vi "HFRR ADV v04 new software.vi"() -> ()   [LabVIEW 2025] (continued)
              n1808 = String Subset(string=w2052, offset (0)=25, length (rest)=9 ("length (rest)")) -> (substring=w2057:string)
              n1809 = String Subset(string=w2052, offset (0)=45, length (rest)=9 ("length (rest)")) -> (substring=w2065:string)
              n1810 = String Subset(string=w2052, offset (0)=0, length (rest)=14 ("length (rest)")) -> (substring=w2080:string)
              n1811 = String Subset(string=w2052, offset (0)=15, length (rest)=9 ("length (rest)")) -> (substring=w2083:string)
              n1812 = String Subset(string=w2052, offset (0)=65, length (rest)=9 ("length (rest)")) -> (substring=w2069:string)
              n1813 = Fract/Exp String To Number(string=w2055) -> (number=w2051:dbl)  [unwired: 3 in, 1 out]
              n1814 = Fract/Exp String To Number(string=w2077) -> (number=w2075:dbl)  [unwired: 3 in, 1 out]
              n1815 = Fract/Exp String To Number(string=w2063) -> (number=w2060:dbl)  [unwired: 3 in, 1 out]
              n1816 = Fract/Exp String To Number(string=w2057) -> (number=w2056:dbl)  [unwired: 3 in, 1 out]
              n1817 = Fract/Exp String To Number(string=w2065) -> (number=w2064:dbl)  [unwired: 3 in, 1 out]
              n1818 = Fract/Exp String To Number(string=w2080) -> (number=w2076:dbl)  [unwired: 3 in, 1 out]
              n1819 = Fract/Exp String To Number(string=w2083) -> (number=w2074:dbl)  [unwired: 3 in, 1 out]
              n1820 = Fract/Exp String To Number(string=w2069) -> (number=w2072:dbl)  [unwired: 3 in, 1 out]
              n1821 = Add(x=w2072, y=0.0) -> (x+y=w2068:dbl)
            }
            n1822 = for {
              N: w1960 -> [_]
              tunnel: w1967 -> [w2015]
              tunnel: w1966 -> [w2014]
              tunnel: [w2004] -> w1920 mode=indexing
              tunnel: [w2003] -> w1913 mode=indexing
              tunnel: w1957 -> [_]
              tunnel: [w1992] -> w1918 mode=indexing
              tunnel: [w1997] -> w1915 mode=indexing
              tunnel: [w1993] -> w1905 mode=indexing
              tunnel: [w1988] -> w1880 mode=indexing
              tunnel: [w1984] -> w1861 mode=indexing
              tunnel: [w1979] -> w1821 mode=indexing
              (unwired) 1.0 ("x")
              (unwired) TRUE ("line mode (F)")
              n1823 = Read from Text File "Read File"(file (use dialog)=w2015, error in=w2014) -> (text=w1980:string)  [unwired: 2 in, 3 out]
              n1824 = local write "String 12"(w1980) -> ()
              n1825 = String Subset(string=w1980, offset (0)=85, length (rest)=9 ("length (rest)")) -> (substring=w1982:string)
              n1826 = String Subset(string=w1980, offset (0)=35, length (rest)=9 ("length (rest)")) -> (substring=w2005:string)
              n1827 = String Subset(string=w1980, offset (0)=55, length (rest)=9 ("length (rest)")) -> (substring=w1990:string)
              n1828 = String Subset(string=w1980, offset (0)=25, length (rest)=9 ("length (rest)")) -> (substring=w1986:string)
              n1829 = String Subset(string=w1980, offset (0)=45, length (rest)=9 ("length (rest)")) -> (substring=w1995:string)
              n1830 = String Subset(string=w1980, offset (0)=15, length (rest)=9 ("length (rest)")) -> (substring=w2011:string)
              n1831 = String Subset(string=w1980, offset (0)=0, length (rest)=14 ("length (rest)")) -> (substring=w2008:string)
              n1832 = String Subset(string=w1980, offset (0)=65, length (rest)=9 ("length (rest)")) -> (substring=w1998:string)
              n1833 = Fract/Exp String To Number(string=w1982) -> (number=w1979:dbl)  [unwired: 3 in, 1 out]
              n1834 = Fract/Exp String To Number(string=w2005) -> (number=w2003:dbl)  [unwired: 3 in, 1 out]
              n1835 = Fract/Exp String To Number(string=w1990) -> (number=w1988:dbl)  [unwired: 3 in, 1 out]
              n1836 = Fract/Exp String To Number(string=w1986) -> (number=w1984:dbl)  [unwired: 3 in, 1 out]
              n1837 = Fract/Exp String To Number(string=w1995) -> (number=w1993:dbl)  [unwired: 3 in, 1 out]
              n1838 = Fract/Exp String To Number(string=w2011) -> (number=w1992:dbl)  [unwired: 3 in, 1 out]
              n1839 = Fract/Exp String To Number(string=w2008) -> (number=w2004:dbl)  [unwired: 3 in, 1 out]
              n1840 = Fract/Exp String To Number(string=w1998) -> (number=w2001:dbl)  [unwired: 3 in, 1 out]
              n1841 = Add(x=w2001, y=0.0) -> (x+y=w1997:dbl)
            }
            n1842 = Delete From Array(array=w1863, index=0) -> (array with subset deleted=w1836:dbl[])  [unwired: 1 in, 1 out]
            n1843 = Delete From Array(array=w1926, index=0) -> (array with subset deleted=w1899:dbl[])  [unwired: 1 in, 1 out]
            n1844 = Delete From Array(array=w1906, index=0) -> (array with subset deleted=w1894:dbl[])  [unwired: 1 in, 1 out]
            n1845 = Delete From Array(array=w1924, index=0) -> (array with subset deleted=w1925:dbl[])  [unwired: 1 in, 1 out]
            n1846 = call-poly <vilib>:"Mean.vi"("X"=w1836) -> ("mean"=→"КОФ2 4":dbl)  [unwired: 1 out]
            n1847 = call-poly <vilib>:"Mean.vi"("X"=w1899) -> ("mean"=→"КОФ3":dbl)  [unwired: 1 out]
            n1848 = call-poly <vilib>:"Mean.vi"("X"=w1894) -> ("mean"=→"CP3":dbl)  [unwired: 1 out]
            n1849 = Delete From Array(array=w1888, index=0) -> (array with subset deleted=w1815:dbl[])  [unwired: 1 in, 1 out]
            n1850 = Delete From Array(array=w1827, index=0) -> (array with subset deleted=w1814:dbl[])  [unwired: 1 in, 1 out]
            n1851 = Delete From Array(array=w1867, index=0) -> (array with subset deleted=w1838:dbl[])  [unwired: 1 in, 1 out]
            n1852 = Delete From Array(array=w1945, index=0) -> (array with subset deleted=w1900:dbl[])  [unwired: 1 in, 1 out]
            n1853 = Delete From Array(array=w1911, index=0) -> (array with subset deleted=w1896:dbl[])  [unwired: 1 in, 1 out]
            "array w/ subset deleted" <- w1896
            n1854 = Delete From Array(array=w1942, index=0) -> (array with subset deleted=w1943:dbl[])  [unwired: 1 in, 1 out]
            n1855 = call-poly <vilib>:"Mean.vi"("X"=w1838) -> ("mean"=→"КОФ2 2":dbl)  [unwired: 1 out]
            n1856 = call-poly <vilib>:"Mean.vi"("X"=w1900) -> ("mean"=→"КОФ1":dbl)  [unwired: 1 out]
            n1857 = Bundle "Bundle"(w1815, w1814) -> (w1820:cluster{dbl[], dbl[]})  [unwired: 1 in]
            n1858 = Bundle "Bundle"(w1815, w1943) -> (w1807:cluster{dbl[], dbl[]})  [unwired: 1 in]
            n1859 = Delete From Array(array=w1822, index=0) -> (array with subset deleted=w1810:dbl[])  [unwired: 1 in, 1 out]
            n1860 = Delete From Array(array=w1823, index=0) -> (array with subset deleted=w1812:dbl[])  [unwired: 1 in, 1 out]
            n1861 = Delete From Array(array=w1933, index=0) -> (array with subset deleted=w1934:dbl[])  [unwired: 1 in, 1 out]
            n1862 = Delete From Array(array=w1821, index=0) -> (array with subset deleted=w1808:dbl[])  [unwired: 1 in, 1 out]
            n1863 = Delete From Array(array=w1915, index=0) -> (array with subset deleted=w1916:dbl[])  [unwired: 1 in, 1 out]
            n1864 = Delete From Array(array=w1940, index=0) -> (array with subset deleted=w1846:dbl[])  [unwired: 1 in, 1 out]
            n1865 = Delete From Array(array=w1886, index=0) -> (array with subset deleted=w1842:dbl[])  [unwired: 1 in, 1 out]
            n1866 = Delete From Array(array=w1922, index=0) -> (array with subset deleted=w1844:dbl[])  [unwired: 1 in, 1 out]
            n1867 = Delete From Array(array=w1882, index=0) -> (array with subset deleted=w1840:dbl[])  [unwired: 1 in, 1 out]
            n1868 = Delete From Array(array=w1931, index=0) -> (array with subset deleted=w1845:dbl[])  [unwired: 1 in, 1 out]
            n1869 = Delete From Array(array=w1884, index=0) -> (array with subset deleted=w1841:dbl[])  [unwired: 1 in, 1 out]
            n1870 = Delete From Array(array=w1865, index=0) -> (array with subset deleted=w1837:dbl[])  [unwired: 1 in, 1 out]
            n1871 = Delete From Array(array=w1909, index=0) -> (array with subset deleted=w1895:dbl[])  [unwired: 1 in, 1 out]
            n1872 = Delete From Array(array=w1936, index=0) -> (array with subset deleted=w1897:dbl[])  [unwired: 1 in, 1 out]
            n1873 = Delete From Array(array=w1913, index=0) -> (array with subset deleted=w1843:dbl[])  [unwired: 1 in, 1 out]
            n1874 = Delete From Array(array=w1880, index=0) -> (array with subset deleted=w1839:dbl[])  [unwired: 1 in, 1 out]
            n1875 = Delete From Array(array=w1861, index=0) -> (array with subset deleted=w1835:dbl[])  [unwired: 1 in, 1 out]
            n1876 = Delete From Array(array=w1905, index=0) -> (array with subset deleted=w1893:dbl[])  [unwired: 1 in, 1 out]
            n1877 = Delete From Array(array=w1918, index=0) -> (array with subset deleted=w1898:dbl[])  [unwired: 1 in, 1 out]
            n1878 = Delete From Array(array=w1928, index=0) -> (array with subset deleted=w1811:dbl[])  [unwired: 1 in, 1 out]
            n1879 = Delete From Array(array=w1938, index=0) -> (array with subset deleted=w1813:dbl[])  [unwired: 1 in, 1 out]
            n1880 = Delete From Array(array=w1920, index=0) -> (array with subset deleted=w1809:dbl[])  [unwired: 1 in, 1 out]
            n1881 = Bundle "Bundle"(w1815, w1846) -> (w1833:cluster{dbl[], dbl[]})  [unwired: 1 in]
            n1882 = Bundle "Bundle"(w1815, w1900) -> (w1834:cluster{dbl[], dbl[]})  [unwired: 1 in]
            n1883 = Bundle "Bundle"(w1846, w1842) -> (w1848:cluster{dbl[], dbl[]})  [unwired: 1 in]
            n1884 = Bundle "Bundle"(w1811, w1810) -> (w1818:cluster{dbl[], dbl[]})  [unwired: 1 in]
            n1885 = Bundle "Bundle"(w1844, w1840) -> (w1850:cluster{dbl[], dbl[]})  [unwired: 1 in]
            n1886 = Bundle "Bundle"(w1811, w1844) -> (w1954:cluster{dbl[], dbl[]})  [unwired: 1 in]
            n1887 = Bundle "Bundle"(w1811, w1840) -> (w1878:cluster{dbl[], dbl[]})  [unwired: 1 in]
            n1888 = Bundle "Bundle"(w1811, w1899) -> (w1964:cluster{dbl[], dbl[]})  [unwired: 1 in]
            n1889 = Bundle "Bundle"(w1811, w1894) -> (w1902:cluster{dbl[], dbl[]})  [unwired: 1 in]
            n1890 = Bundle "Bundle"(w1811, w1925) -> (w1949:cluster{dbl[], dbl[]})  [unwired: 1 in]
            n1891 = Bundle "Bundle"(w1845, w1841) -> (w1849:cluster{dbl[], dbl[]})  [unwired: 1 in]
            n1892 = Bundle "Bundle"(w1813, w1812) -> (w1819:cluster{dbl[], dbl[]})  [unwired: 1 in]
            n1893 = Bundle "Bundle"(w1813, w1845) -> (w1956:cluster{dbl[], dbl[]})  [unwired: 1 in]
            n1894 = Bundle "Bundle"(w1813, w1841) -> (w1879:cluster{dbl[], dbl[]})  [unwired: 1 in]
            n1895 = Bundle "Bundle"(w1813, w1895) -> (w1903:cluster{dbl[], dbl[]})  [unwired: 1 in]
            n1896 = Bundle "Bundle"(w1813, w1897) -> (w1965:cluster{dbl[], dbl[]})  [unwired: 1 in]
            n1897 = Bundle "Bundle"(w1813, w1934) -> (w1947:cluster{dbl[], dbl[]})  [unwired: 1 in]
            n1898 = Bundle "Bundle"(w1843, w1839) -> (w1851:cluster{dbl[], dbl[]})  [unwired: 1 in]
            n1899 = Bundle "Bundle"(w1809, w1808) -> (w1817:cluster{dbl[], dbl[]})  [unwired: 1 in]
            n1900 = Bundle "Bundle"(w1809, w1843) -> (w1955:cluster{dbl[], dbl[]})  [unwired: 1 in]
            n1901 = Bundle "Bundle"(w1809, w1839) -> (w1877:cluster{dbl[], dbl[]})  [unwired: 1 in]
            n1902 = Bundle "Bundle"(w1809, w1893) -> (w1901:cluster{dbl[], dbl[]})  [unwired: 1 in]
            n1903 = Bundle "Bundle"(w1809, w1898) -> (w1963:cluster{dbl[], dbl[]})  [unwired: 1 in]
            n1904 = Bundle "Bundle"(w1809, w1916) -> (w1948:cluster{dbl[], dbl[]})  [unwired: 1 in]
            n1905 = call-poly <vilib>:"Mean.vi"("X"=w1896) -> ("mean"=→"CP1":dbl)  [unwired: 1 out]
            n1906 = call-poly <vilib>:"Mean.vi"("X"=w1837) -> ("mean"=→"КОФ2 3":dbl)  [unwired: 1 out]
            n1907 = call-poly <vilib>:"Mean.vi"("X"=w1895) -> ("mean"=→"CP2":dbl)  [unwired: 1 out]
            n1908 = call-poly <vilib>:"Mean.vi"("X"=w1897) -> ("mean"=→"КОФ2":dbl)  [unwired: 1 out]
            n1909 = call-poly <vilib>:"Mean.vi"("X"=w1835) -> ("mean"=→"КОФ2 5":dbl)  [unwired: 1 out]
            n1910 = call-poly <vilib>:"Mean.vi"("X"=w1893) -> ("mean"=→"CP4":dbl)  [unwired: 1 out]
            n1911 = call-poly <vilib>:"Mean.vi"("X"=w1898) -> ("mean"=→"КОФ4":dbl)  [unwired: 1 out]
            n1912 = Bundle "Bundle"(w1815, w1842) -> (w1806:cluster{dbl[], dbl[]})  [unwired: 1 in]
            n1913 = Bundle "Bundle"(w1815, w1896) -> (w1829:cluster{dbl[], dbl[]})  [unwired: 1 in]
            n1914 = Build Array "Build Array"(w1806, w1829) -> (w1832:cluster{dbl[], dbl[]}[])
            "XY Graph 17" <- w1832
            n1915 = Build Array "Build Array"(w1820, w1819, w1818, w1817) -> (→"Frequency ( Hz )":cluster{dbl[], dbl[]}[])
            n1916 = Build Array "Build Array"(w1848, w1849, w1850, w1851) -> (→"Air Temp ( °C ) vs Humidity ( % RH )":cluster{dbl[], dbl[]}[])
            n1917 = Build Array "Build Array"(w1833, w1956, w1954, w1955) -> (→"Air Temperature  ( °C )":cluster{dbl[], dbl[]}[])
            n1918 = Build Array "Build Array"(w1806, w1879, w1878, w1877) -> (→"Humidity ( %RH )":cluster{dbl[], dbl[]}[])
            n1919 = Build Array "Build Array"(w1834, w1965, w1964, w1963) -> (→"Coefficient Of Friction":cluster{dbl[], dbl[]}[])
            n1920 = Build Array "Build Array"(w1829, w1903, w1902, w1901) -> (→"Sample Temperature ( °C )":cluster{dbl[], dbl[]}[])
            n1921 = Build Array "Build Array"(w1807, w1947, w1949, w1948) -> (→"XY Graph 13":cluster{dbl[], dbl[]}[])
            n1922 = Bundle "Bundle"(w1815, w1838) -> (w1860:cluster{dbl[], dbl[]})  [unwired: 1 in]
            n1923 = Bundle "Bundle"(w1811, w1836) -> (w1858:cluster{dbl[], dbl[]})  [unwired: 1 in]
            n1924 = Bundle "Bundle"(w1813, w1837) -> (w1859:cluster{dbl[], dbl[]})  [unwired: 1 in]
            n1925 = Bundle "Bundle"(w1809, w1835) -> (w1857:cluster{dbl[], dbl[]})  [unwired: 1 in]
            n1926 = Build Array "Build Array"(w1860, w1859, w1858, w1857) -> (→"Stroke ( mm )":cluster{dbl[], dbl[]}[])
            n1927 = local write "XY Graph 16"(w1832) -> ()
          }
          frame #2 {
          }
          frame #3 {
            n1928 = local write "Numeric 8"(0 ("Numeric 8")) -> ()
            n1929 = local write "Numeric 11"(0 ("Numeric 11")) -> ()
            n1930 = local write "Numeric 12"(0 ("Numeric 12")) -> ()
            n1931 = local write "Numeric 13"(0 ("Numeric 13")) -> ()
            n1932 = property on="OPEN" class="Bool (strict)"("Visible"=TRUE) -> ()  [unwired: 2 in, 2 out]
            n1933 = local read "String Control 2"() -> (w2132:string)
            n1934 = local read "String Control 4"() -> (w2131:string)
            n1935 = local read "String Control 6"() -> (w2130:string)
            n1936 = local read "String Control 8"() -> (w2129:string)
            n1937 = Match Pattern(string=w2132, regular expression="Samples / cycle :- ") -> (after substring=w2146:string)  [unwired: 1 in, 3 out]
            n1938 = Match Pattern(string=w2132, regular expression="Frequency :- ") -> (after substring=w2165:string)  [unwired: 1 in, 3 out]
            n1939 = Match Pattern(string=w2131, regular expression="Samples / cycle :- ") -> (after substring=w2142:string)  [unwired: 1 in, 3 out]
            n1940 = Match Pattern(string=w2131, regular expression="Frequency :- ") -> (after substring=w2160:string)  [unwired: 1 in, 3 out]
            n1941 = Match Pattern(string=w2130, regular expression="Samples / cycle :- ") -> (after substring=w2138:string)  [unwired: 1 in, 3 out]
            n1942 = Match Pattern(string=w2130, regular expression="Frequency :- ") -> (after substring=w2155:string)  [unwired: 1 in, 3 out]
            n1943 = Match Pattern(string=w2129, regular expression="Samples / cycle :- ") -> (after substring=w2134:string)  [unwired: 1 in, 3 out]
            n1944 = Match Pattern(string=w2129, regular expression="Frequency :- ") -> (after substring=w2150:string)  [unwired: 1 in, 3 out]
            n1945 = String Subset(string=w2146, length (rest)=6 ("length (rest)")) -> (substring=w2148:string)  [unwired: 1 in]
            n1946 = String Subset(string=w2165, length (rest)=9 ("length (rest)")) -> (substring=w2167:string)  [unwired: 1 in]
            n1947 = String Subset(string=w2142, length (rest)=6 ("length (rest)")) -> (substring=w2144:string)  [unwired: 1 in]
            n1948 = String Subset(string=w2160, length (rest)=9 ("length (rest)")) -> (substring=w2162:string)  [unwired: 1 in]
            n1949 = String Subset(string=w2138, length (rest)=6 ("length (rest)")) -> (substring=w2140:string)  [unwired: 1 in]
            n1950 = String Subset(string=w2155, length (rest)=9 ("length (rest)")) -> (substring=w2157:string)  [unwired: 1 in]
            n1951 = String Subset(string=w2134, length (rest)=6 ("length (rest)")) -> (substring=w2136:string)  [unwired: 1 in]
            n1952 = String Subset(string=w2150, length (rest)=9 ("length (rest)")) -> (substring=w2152:string)  [unwired: 1 in]
            n1953 = Fract/Exp String To Number(string=w2148) -> (number=w2128:dbl)  [unwired: 3 in, 1 out]
            n1954 = Fract/Exp String To Number(string=w2167) -> (number=w2168:dbl)  [unwired: 3 in, 1 out]
            n1955 = Fract/Exp String To Number(string=w2144) -> (number=w2127:dbl)  [unwired: 3 in, 1 out]
            n1956 = Fract/Exp String To Number(string=w2162) -> (number=w2163:dbl)  [unwired: 3 in, 1 out]
            n1957 = Fract/Exp String To Number(string=w2140) -> (number=w2126:dbl)  [unwired: 3 in, 1 out]
            n1958 = Fract/Exp String To Number(string=w2157) -> (number=w2158:dbl)  [unwired: 3 in, 1 out]
            n1959 = Fract/Exp String To Number(string=w2136) -> (number=w2125:dbl)  [unwired: 3 in, 1 out]
            n1960 = Fract/Exp String To Number(string=w2152) -> (number=w2153:dbl)  [unwired: 3 in, 1 out]
            n1961 = local write "sample1"(w2128) -> ()
            n1962 = local write "freq1"(w2168) -> ()
            n1963 = local write "sample2"(w2127) -> ()
            n1964 = local write "freq2"(w2163) -> ()
            n1965 = local write "sample3"(w2126) -> ()
            n1966 = local write "freq3"(w2158) -> ()
            n1967 = local write "sample4"(w2125) -> ()
            n1968 = local write "freq 4"(w2153) -> ()
          }
        }
      }
    }
    n1969 = case shown="True" w1617 {
      selector: w1617 -> [_ w1745]
      frame False {
      }
      frame True {
        n1970 = Not(x=w1745) -> (.not. x?=w1741:bool)
        n1971 = local write "service 3"(w1741) -> ()
        n1972 = local write "OPEN 6"(w1741) -> ()
        n1973 = call <vilib>:"System Exec.vi"("wait until completion? (T)"=TRUE, "command line"="C:\\LAB-IQ\\Scar View.exe") -> ("error out"=→"error out 5":errorcluster)  [unwired: 6 in, 3 out]
      }
    }
    n1974 = case shown="\"Acquire\", Default" w1628 {
      frame "Acquire", Default {
        w2641 = 0.2 ("y")
        w2646 = 1.0 ("y")
        w2647 = 0.8 ("y")
        # "Elapsed time\ncof\nstroke\nAir temp\nTemp\nHumidity"
        n1975 = disable-structure shown="Disabled" {
          frame Disabled {
            n1976 = local read "Flag"() -> (w2664:dbl)
            n1977 = local read "RUN"() -> (w2661:bool)
            n1978 = Not(x=w2661) -> (.not. x?=w2660:bool)
            n1979 = Equal?(x=w2664, y=10.0) -> (x = y?=w2662:bool)
            n1980 = And(x=w2662, y=w2660) -> (x .and. y?=w2659:bool)
            n1981 = case shown="True" w2659 {
              frame False {
              }
              frame True {
                w2665 = FALSE ("Heater Button")
                n1982 = local write "Humidity"(w2665) -> ()
                n1983 = local write "Heater Button"(w2665) -> ()
              }
            }
          }
          frame Enabled {
          }
        }
        n1984 = disable-structure shown="Disabled" {
          frame Disabled {
            n1985 = case shown="True" {
              selector: _ -> [_ _]
              frame False {
              }
              frame True {
                w2756 = TRUE ("Heater")
                n1986 = local write "Humidity"(w2756) -> ()
                n1987 = local write "Heater Button"(w2756) -> ()
                n1988 = local read "TEST STANDARD"() -> (w2759:T3)
                n1989 = local read "TEST STANDARD"() -> (w2754:T3)
                n1990 = Equal?(x=w2759, y=enum16{"ASTM D6079", "ISO 12156", "Custom"}."ISO 12156" ("Test Standard")) -> (x = y?=w2757:bool)
                n1991 = Equal?(x=w2754, y=enum16{"ASTM D6079", "ISO 12156", "Custom"}."ASTM D6079" ("Test Standard")) -> (x = y?=w2753:bool)
                n1992 = case shown="True" w2757 {
                  frame False {
                  }
                  frame True {
                    n1993 = local write "Heater"(TRUE ("Heater")) -> ()
                    n1994 = local write "airtempflg"(FALSE ("airtempflg")) -> ()
                  }
                }
                n1995 = case shown="True" w2753 {
                  frame False {
                  }
                  frame True {
                    n1996 = local write "Heater"(FALSE ("Heater")) -> ()
                    n1997 = local write "airtempflg"(TRUE ("airtempflg")) -> ()
                  }
                }
              }
            }
          }
          frame Enabled {
          }
        }
        n1998 = stacked-sequence {
          frame #0 {
            n1999 = case shown="True" "RST FF" {
              frame False {
              }
              frame True {
                w2822 = 0.0 ("X Scale.Range:Maximum")
                n2000 = property on="Frictional Force ( N )" class="WFChart (strict)"("XScale.Maximum"=600.0 ("X Scale.Range:Maximum"), "XScale.Minimum"=w2822, "YScale.Maximum"=10.0 ("Y Scale.Range:Maximum"), "YScale.Minimum"=w2822) -> ()  [unwired: 2 in, 2 out]
              }
            }
          }
          frame #1 {
            n2001 = case shown="True" "RST TEMP" {
              frame False {
              }
              frame True {
                n2002 = property on="Temperature ( Deg C )" class="WFChart (strict)"("XScale.Minimum"=0.0 ("X Scale.Range:Minimum"), "XScale.Maximum"=600.0 ("X Scale.Range:Maximum"), "YScale.Minimum"=0.0 ("Y Scale.Range:Minimum"), "YScale.Maximum"=100.0 ("Y Scale.Range:Maximum")) -> ()  [unwired: 2 in, 2 out]
              }
            }
          }
          frame #2 {
            n2003 = case shown="True" "RSTCOF" {
              frame False {
              }
              frame True {
                n2004 = property on="Coefficient of Friction" class="WFChart (strict)"("XScale.Minimum"=0.0 ("X Scale.Range:Minimum"), "XScale.Maximum"=600.0 ("X Scale.Range:Maximum"), "YScale.Maximum"=1.0 ("X Scale.Range:Minimum"), "YScale.Minimum"=0.0 ("X Scale.Range:Minimum")) -> ()  [unwired: 2 in, 2 out]
              }
            }
          }
          frame #3 {
            n2005 = case shown="True" "RSTCOF 2" {
              frame False {
              }
              frame True {
                (unwired) 100.0 ("Y Scale.Range:Maximum")
                (unwired) 0.0 ("Y Scale.Range:Minimum")
                (unwired) 600.0 ("X Scale.Range:Maximum")
                (unwired) 0.0 ("X Scale.Range:Minimum")
              }
            }
          }
          frame #4 {
            n2006 = case shown="True" "RSTCOF 3" {
              frame False {
              }
              frame True {
                n2007 = property on="Electrical Contact Resistance ( % )" class="WFChart (strict)"("XScale.Minimum"=0.0 ("X Scale.Range:Minimum"), "XScale.Maximum"=600.0 ("X Scale.Range:Maximum"), "YScale.Minimum"=0.0 ("Y Scale.Range:Minimum"), "YScale.Maximum"=100.0 ("Y Scale.Range:Maximum")) -> ()  [unwired: 2 in, 2 out]
              }
            }
          }
        }
        n2008 = disable-structure shown="Disabled" {
          frame Disabled {
            n2009 = case shown="True" {
              selector: _ -> [_ _]
              frame False {
              }
              frame True {
                n2010 = local read "zflag 2"() -> (w2723:dbl)
                n2011 = local read "yflag"() -> (w2725:dbl)
                n2012 = Equal?(x=w2725, y=2.0 ("tflag")) -> (x = y?=w2727:bool)
                n2013 = Equal?(x=w2723, y=3.0 ("tflag")) -> (x = y?=w2726:bool)
                n2014 = And(x=w2727, y=w2726) -> (x .and. y?=w2721:bool)
                n2015 = case shown="True" w2721 {
                  frame False {
                  }
                  frame True {
                    w2752 = 0.0 ("zflag")
                    n2016 = local write "zflag"(w2752) -> ()
                    n2017 = local write "zflag 2"(w2752) -> ()
                    n2018 = Delete(path (use dialog)=path "C:/LAB-IQ-NXT/WO 2449 TT.sig" ("file path (dialog if empty)")) -> (deleted path=w2751:path)  [unwired: 4 in, 2 out]
                    n2019 = Delete(path (use dialog)=path "C:/LAB-IQ-NXT/WO 2449 TRH.sig" ("file path (dialog if empty)")) -> (deleted path=w2746:path)  [unwired: 4 in, 2 out]
                    n2020 = local read "SEN.RUN HRS"() -> (w2738:dbl)
                    n2021 = local read "SENSOR TIME"() -> (w2736:dbl)
                    n2022 = call <vilib>:"compatOverwrite.vi"("overwrite (F)"=TRUE) -> ("overwrite?"=w2728:T23)
                    n2023 = call <vilib>:"compatOverwrite.vi"("overwrite (F)"=TRUE) -> ("overwrite?"=w2732:T23)
                    n2024 = local read "Total No. of Tests"() -> (w2739:dbl)
                    n2025 = Add(x=w2736, y=w2738) -> (x+y=w2737:dbl)
                    "SEN.RUN HRS" <- w2737
                    n2026 = Open/Create/Replace File(file path (use dialog)=w2751, operation (0:open)=w2728) -> (refnum out=w2729:refnum<file>, error out=w2730:errorcluster)  [unwired: 4 in, 1 out]
                    n2027 = Open/Create/Replace File(file path (use dialog)=w2746, operation (0:open)=w2732) -> (refnum out=w2733:refnum<file>, error out=w2734:errorcluster)  [unwired: 4 in, 1 out]
                    n2028 = Deny Access(4:w2730, 6:T21."deny none" ("deny mode (2)"), 7:w2729) -> (3:w2750:refnum<file>)  [unwired: 1 out]
                    n2029 = Deny Access(4:w2734, 6:T21."deny none" ("deny mode (2)"), 7:w2733) -> (3:w2742:refnum<file>)  [unwired: 1 out]
                    n2030 = Number To Decimal String(number=w2739) -> (decimal integer string=w2747:string)  [unwired: 1 in]
                    n2031 = Number To Decimal String(number=w2737) -> (decimal integer string=w2743:string)  [unwired: 1 in]
                    n2032 = Write to Binary File(file (use dialog)=w2750, data=w2747, 5:FALSE ("prepend array or string size? (T)")) -> ()  [unwired: 3 in, 3 out]
                    n2033 = Write to Binary File(file (use dialog)=w2742, data=w2743, 5:FALSE ("prepend array or string size? (T)")) -> ()  [unwired: 3 in, 3 out]
                  }
                }
              }
            }
          }
          frame Enabled {
          }
        }
        n2034 = local read "RUN"() -> (w2650:bool)
        n2035 = local read "run replace"() -> (w2654:bool)
        n2036 = local read "run replace"() -> (w2653:bool)
        n2037 = case shown="True" w2650 {
          frame False {
            n2038 = local write "run replace"(FALSE ("run replace")) -> ()
          }
          frame True {
            "run replace" <- TRUE ("run replace")
          }
        }
        n2039 = local read "RUN"() -> (w2658:bool)
        n2040 = local read "Set Temp"() -> (w2620:dbl)
        n2041 = local read "SetTemp"() -> (w2622:dbl)
        n2042 = case shown="False" w2658 {
          tunnel: [FALSE ("TEST RUNNING") TRUE ("TEST RUNNING")] -> w2657
          frame False {
            w2841 = 0.0 ("Flag")
            n2043 = local write "Elapsed time"(0.0 ("elapsedtime")) -> ()
            n2044 = local write "Time Remaining"(w2841) -> ()
            n2045 = local write "Flag"(w2841) -> ()
            n2046 = local write "Remaining Time"(w2841) -> ()
          }
          frame True {
            n2047 = local write "Flag"(10.0 ("Flag")) -> ()
          }
        }
        n2048 = case shown="False" w2654 {
          frame False {
            n2049 = local read "zflag"() -> (→"zflag 2":dbl)
            n2050 = local write "yflag"(2.0 ("tflag")) -> ()
            n2051 = local write "FLAG 4"(0.0 ("FLAG")) -> ()
          }
          frame True {
            n2052 = local write "yflag"(1.0 ("tflag")) -> ()
            n2053 = local write "zflag"(3.0 ("zflag")) -> ()
          }
        }
        n2054 = local read "acq 2"() -> (w2652:bool)
        n2055 = local read "AIR TEMP"() -> (w2615:dbl)
        n2056 = local read "Amb temp"() -> (w2619:dbl)
        n2057 = case shown="True" "Save & Continue" {
          frame False {
          }
          frame True {
            "acq 2" <- TRUE ("acq 2")
          }
        }
        n2058 = local read "Set Rh"() -> (w2621:dbl)
        n2059 = Add(x=w2622, y=w2647) -> (x+y=w2648:dbl)
        n2060 = Subtract(x=w2622, y=w2647) -> (x-y=w2649:dbl)
        n2061 = Add(x=w2620, y=w2641) -> (x+y=w2642:dbl)
        n2062 = Subtract(x=w2620, y=w2641) -> (x-y=w2643:dbl)
        n2063 = And(x=w2652, y=w2653) -> (x .and. y?=w2651:bool)
        n2064 = Greater Or Equal?(x=w2615, y=15.0) -> (x >= y?=w2616:bool)
        "powstat" <- w2616
        n2065 = local read "Humidity ( %RH )"() -> (w2618:dbl)
        n2066 = case shown="True" "Save & Continue" {
          frame False {
          }
          frame True {
            n2067 = while {
              tunnel: "0123456789abcdefghijklmnopqrstuvwxyzABCDEFGHIJKLMNOPQRSTUVWXYZ" ("string 2") -> [w2812]
              shift-right: [w2810] -> w2805
              shift-left: "" -> [w2809]
              i -> [w2819]
              stop <- w2818 stop-if-true
              n2068 = Random Number (0-1)() -> (number: 0 to 1=w2813:dbl)
              n2069 = Multiply(x=w2813, y=62.0) -> (x*y=w2815:dbl)
              n2070 = Decrement(x="Length") -> (x-1=w2808:i16)
              n2071 = To Word Integer(number=w2815) -> (16bit integer=w2816:i16)
              n2072 = String Subset(string=w2812, offset (0)=w2816, length (rest)=1 ("length (rest)")) -> (substring=w2811:string)
              n2073 = Greater Or Equal?(x=w2819, y=w2808) -> (x >= y?=w2818:bool)
              n2074 = Concatenate Strings(w2811, w2809) -> (w2810:string)
            }
            n2075 = local write "UUID"(w2805) -> ()
          }
        }
        n2076 = In Range and Coerce(upper limit=w2648, x=w2619, lower limit=w2649) -> (In Range?=w2638:bool)  [unwired: 1 out]
        n2077 = Add(x=w2621, y=w2646) -> (x+y=w2645:dbl)
        n2078 = Subtract(x=w2621, y=w2646) -> (x-y=w2644:dbl)
        n2079 = local read "TEMP"() -> (w2617:dbl)
        n2080 = case shown="True" "Save & Continue" {
          frame False {
          }
          frame True {
            n2081 = local read "Operator ID"() -> (w3116:string)
            n2082 = local read "FILE"() -> (w3122:string)
            n2083 = String Length(string=w3122) -> (length=w3120:i32)
            n2084 = String Length(string=w3116) -> (length=w3117:i32)
            n2085 = Greater?(x=w3120, y=0) -> (0:w3119:bool)
            n2086 = Greater?(x=w3117, y=0) -> (0:w3115:bool)
            n2087 = And(x=w3119, y=w3115) -> (x .and. y?=w3114:bool)
            n2088 = case shown="True" w3114 {
              frame False {
                n2089 = stacked-sequence {
                  frame #0 {
                    n2090 = One Button Dialog(message="Please Enter a File Name and Operator ID to save data !", button name ("OK")="Ok") -> ()  [unwired: 1 out]
                  }
                  frame #1 {
                    n2091 = local write "Save & Continue"(FALSE ("OK Button")) -> ()
                  }
                }
                n2092 = local write "Save & Continue"(FALSE ("OK Button")) -> ()
              }
              frame True {
                n2093 = stacked-sequence {
                  frame #0 {
                    n2094 = local read "FILE"() -> (w3128:string)
                    n2095 = call "file check.vi"("file name in"=w3128) -> ("file name out"=w3127:string)  [unwired: 9 in, 1 out]
                    n2096 = call <vilib>:"Application Directory.vi"() -> ("Application Directory"=w3138:path)
                    n2097 = Build Path(base path=w3138, name or relative path="data") -> (appended path=w3137:path)
                    n2098 = call <vilib>:"Trim Whitespace.vi"("string"=w3127) -> ("trimmed string"=w3135:string)  [unwired: 1 in]
                    n2099 = call <vilib>:"Trim Whitespace.vi"("string"=w3127) -> ("trimmed string"=w3136:string)  [unwired: 1 in]
                    n2100 = List Folder(path=w3137) -> (folder names=w3133:string[])  [unwired: 3 in, 3 out]
                    n2101 = Match Pattern(string=w3135, regular expression="_(") -> (before substring=w3132:string)  [unwired: 1 in, 3 out]
                    n2102 = for {
                      tunnel: w3133 -> [w3147] mode=indexing
                      tunnel: w3132 -> [w3145]
                      shift-right: [w3143] -> w3130
                      shift-left: bool[] [] -> [w3144]
                      n2103 = Match Pattern(string=w3147, regular expression="_(") -> (before substring=w3146:string)  [unwired: 1 in, 3 out]
                      n2104 = Equal?(x=w3146, y=w3145) -> (x = y?=w3142:bool)
                      n2105 = case shown="True" w3142 {
                        tunnel: w3142 -> [_ w3150]
                        tunnel: w3144 -> [w3149 w3152]
                        tunnel: [w3149 w3151] -> w3143
                        frame False {
                        }
                        frame True {
                          n2106 = Insert Into Array(array=w3152, new element=w3150) -> (w3151:bool[])  [unwired: 1 in]
                        }
                      }
                    }
                    n2107 = Equal?(x=w3133, y=w3132) -> (x = y?=w3141:bool[])
                    n2108 = Or Array Elements(Boolean array=w3141) -> (logical OR=w3140:bool)
                    n2109 = Array Size(array=w3130) -> (size(s)=w3129:i32)
                    n2110 = case shown="True" w3140 {
                      tunnel: w3136 -> [_ w3160]
                      tunnel: w3129 -> [_ w3153]
                      frame False {
                      }
                      frame True {
                        n2111 = Number To Decimal String(number=w3153) -> (decimal integer string=w3156:string)  [unwired: 1 in]
                        n2112 = Search/Split String(string=w3160, search string/char (-)="_(" ("regular expression")) -> (substring before match=w3158:string)  [unwired: 1 in, 2 out]
                        n2113 = Concatenate Strings(w3158, "_(" ("regular expression"), w3156, ")" ("regular expression")) -> (w3154:string)
                        n2114 = local write "FILE"(w3154) -> ()
                      }
                    }
                  }
                  frame #1 {
                    w3162 = 0.0
                    w3175 = cluster{"y":dbl, dbl, "y":dbl}[] [] ("History Data")
                    w3176 = FALSE ("Heater Button")
                    (unwired) ")!" ("string")
                    (unwired) ")" ("string")
                    w3174 = dbl[] [] ("History Data")
                    w3180 = "\r"
                    # "C:\\WinDucom\\Data\\"
                    # "C:\\LAB-IQ-NXT\\data"
                    n2115 = local write "Humidity ( %RH )"(w3162) -> ()
                    n2116 = local write "Frequency ( Hz )"(w3162) -> ()
                    n2117 = local write "Stroke 3"(w3162) -> ()
                    n2118 = local write "speedop"(0.0 ("PIDclk 2")) -> ()
                    n2119 = local write "Set Temp 2"(65.0 ("Set Temp 2")) -> ()
                    n2120 = local write "AIR TEMP"(w3162) -> ()
                    n2121 = local write "clk"(0.0 ("clk")) -> ()
                    n2122 = local write "Stroke 4"(w3162) -> ()
                    n2123 = local write "COF 2"(w3162) -> ()
                    n2124 = local write "TEMP"(w3162) -> ()
                    n2125 = local write "ecr 3"(w3162) -> ()
                    n2126 = local write "FF 3"(w3162) -> ()
                    n2127 = local write "FF 2"(w3162) -> ()
                    n2128 = property on="Humidity ( %RH )" class="WFChart (strict)"("History Data"=w3174) -> ()  [unwired: 2 in, 2 out]
                    n2129 = property on="Coefficient of Friction" class="WFChart (strict)"("History Data"=w3174) -> ()  [unwired: 2 in, 2 out]
                    n2130 = property on="Coefficient of Friction" class="WFChart (strict)"("History Data"=w3174) -> ()  [unwired: 2 in, 2 out]
                    n2131 = property on="Frictional Force ( N )" class="WFChart (strict)"("History Data"=w3174) -> ()  [unwired: 2 in, 2 out]
                    n2132 = property on="Electrical Contact Resistance ( % )" class="WFChart (strict)"("History Data"=w3174) -> ()  [unwired: 2 in, 2 out]
                    n2133 = property on="Electrical Contact Resistance ( % )" class="WFChart (strict)"("History Data"=w3174) -> ()  [unwired: 2 in, 2 out]
                    n2134 = property on="Temperature ( Deg C )" class="WFChart (strict)"("History Data"=w3174) -> ()  [unwired: 2 in, 2 out]
                    n2135 = property on="Frictional Force ( N )" class="WFChart (strict)"("History Data"=w3174) -> ()  [unwired: 2 in, 2 out]
                    n2136 = property on="Coefficient of Friction" class="WFChart (strict)"("History Data"=w3174) -> ()  [unwired: 2 in, 2 out]
                    n2137 = property on="Frictional Force ( N )" class="WFChart (strict)"("History Data"=w3174) -> ()  [unwired: 2 in, 2 out]
                    n2138 = property on="Electrical Contact Resistance ( % )" class="WFChart (strict)"("History Data"=w3174) -> ()  [unwired: 2 in, 2 out]
                    n2139 = property on="Temperature ( Deg C )" class="WFChart (strict)"("History Data"=w3174) -> ()  [unwired: 2 in, 2 out]
                    n2140 = property on="Humidity ( %RH )" class="WFChart (strict)"("History Data"=w3174) -> ()  [unwired: 2 in, 2 out]
                    n2141 = property on="Stroke ( mm )" class="WFChart (strict)"("History Data"=w3175) -> ()  [unwired: 2 in, 2 out]
                    n2142 = property on="Stroke ( mm )" class="WFChart (strict)"("History Data"=w3175) -> ()  [unwired: 2 in, 2 out]
                    n2143 = local write "Humidity"(w3176) -> ()
                    n2144 = local write "Heater Button"(w3176) -> ()
                    n2145 = local read "FILE"() -> (w3170:string)
                    n2146 = disable-structure shown="Enabled" {
                      disable-tunnel: [w3215 _] -> w3161
                      frame Enabled {
                        n2147 = local read "NORMAL LOAD"() -> (w3215:dbl)
                      }
                      frame Disabled {
                      }
                    }
                    n2148 = call "file check.vi"("file name in"=w3170) -> ("error out"=w3173:errorcluster, "file name out"=w3167:string)  [unwired: 9 in]
                    n2149 = call "FILE PATH CREATION.vi"("error in"=w3173, "FILE NAME :"=w3167) -> ("FILE OUT"=w3166:path)  [unwired: 8 in, 1 out]
                    n2150 = Concatenate Strings(w3167, ".dgf" ("Substring")) -> (w3172:string)
                    n2151 = Concatenate Strings(w3167, ".duf" ("Substring")) -> (w3168:string)
                    n2152 = Multiply(x=w3161, y=1.0) -> (x*y=w3194:dbl)
                    n2153 = Build Path(base path=w3166, name or relative path=w3172) -> (appended path=w3165:path)
                    n2154 = Build Path(base path=w3166, name or relative path=w3168) -> (appended path=w3164:path)
                    n2155 = Number To Fractional String(number=w3194, width (-)=i16 5, precision (6)=i16 2) -> (F-format string=w3202:string)  [unwired: 1 in]
                    n2156 = local read "Fuel Discription :"() -> (w3190:string)
                    n2157 = local read "Batch Ref Num :"() -> (w3178:string)
                    n2158 = Get Date/Time String(date format (0)=enum16{"short", "long", "abbreviated"}."short") -> (date string=w3213:string, time string=w3210:string)  [unwired: 2 in]
                    n2159 = local read "Remarks :"() -> (w3189:string)
                    n2160 = Concatenate Strings("Load :- " ("Substring"), w3202, " grams ," ("Substring")) -> (w3201:string)
                    n2161 = local read "String 41"() -> (w3181:string)
                    n2162 = Concatenate Strings(w3190) -> (w3191:string)
                    n2163 = Concatenate Strings(w3178) -> (w3177:string)
                    n2164 = Concatenate Strings("tested by") -> (w3185:string)
                    n2165 = Concatenate Strings("(" ("Substring"), w3213, ")" ("Substring"), w3210) -> (w3183:string)
                    "concatenated string" <- w3183
                    n2166 = Concatenate Strings(w3189, "," ("string")) -> (w3188:string)
                    n2167 = Concatenate Strings("  TIME;      COF;       STROKE;     AIR TEMP;  TEMP;  HUMIDITY;  ECR; PID-OUT; FREQUENCY" ("Substring"), "\r") -> (w3197:string)
                    n2168 = Concatenate Strings(w3181, w3180, "Fuel Discription :-" ("Substring"), w3191, w3180, w3201, w3180, "Batch Ref Num :-" ("Substring"), w3177, w3180, " Remarks :- " ("Substring"), w3188, w3180, " Date :- " ("Substring"), w3183, w3180, "Tested By :-" ("Substring"), w3185) -> (w3195:string)
                    "REMARKS" <- w3195
                    n2169 = call <vilib>:"Write Characters To File.vi"("append to file? (new file:F)"=FALSE, "character string"=w3197, "file path (dialog if empty)"=w3165) -> ()  [unwired: 2 in, 1 out]
                    n2170 = call <vilib>:"Write Characters To File.vi"("append to file? (new file:F)"=FALSE, "character string"=w3195, "file path (dialog if empty)"=w3164) -> ()  [unwired: 2 in, 1 out]
                  }
                  frame #2 {
                    n2171 = local write "Cycles elapsed"(0 ("Cycles elapsed")) -> ()
                    n2172 = local write "cyclecount"(0 ("cyclecount")) -> ()
                    n2173 = local write "Save & Continue"(FALSE ("OK")) -> ()
                    n2174 = local write "autostrtflg"(TRUE ("autostrtflg")) -> ()
                    n2175 = local write "Save"(FALSE ("Save")) -> ()
                    n2176 = Get Date/Time In Seconds() -> (seconds since 1Jan1904=w3220:timestamp)
                    n2177 = To Double Precision Float(number=w3220) -> (double precision float=w3219:dbl)
                    n2178 = local write "acq timer"(w3219) -> ()
                    n2179 = One Button Dialog(message="Please ensure sample is mounted properly and machine is ready in all aspects for testing !", button name ("OK")="Ok") -> ()  [unwired: 1 out]
                  }
                  frame #3 {
                    n2180 = stacked-sequence {
                      frame #0 {
                        n2181 = local write "Main Dashboard Buttons"(T1."Dashboard" ("Main Dashboard Buttons")) -> ()
                        n2182 = local write "Main Tab"(T2."Acquire" ("Main Tab")) -> ()
                      }
                      frame #1 {
                        n2183 = local write "EVENT LOG"("" ("EVENT LOG")) -> ()
                      }
                      frame #2 {
                        n2184 = Wait (ms)(milliseconds to wait=u32 50) -> ()  [unwired: 1 out]
                      }
                      frame #3 {
                        n2185 = disable-structure shown="Disabled" {
                          frame Disabled {
                            n2186 = local read "EVENT LOG"() -> (w3232:string)
                            n2187 = call "Event Log.vi"("Content"="Test Details", "EVENT LOG"=w3232) -> ("EVENT LOG"=w3231:string)  [unwired: 8 in, 1 out]
                            n2188 = local write "EVENT LOG"(w3231) -> ()
                          }
                          frame Enabled {
                          }
                        }
                      }
                      frame #4 {
                        n2189 = Wait (ms)(milliseconds to wait=u32 50) -> ()  [unwired: 1 out]
                      }
                      frame #5 {
                        n2190 = local read "FILE"() -> (w3234:string)
                        n2191 = Concatenate Strings("File Name :" ("Content"), w3234) -> (w3235:string)
                        n2192 = local read "EVENT LOG"() -> (w3238:string)
                        n2193 = call "Event Log.vi"("Content"=w3235, "EVENT LOG"=w3238) -> ("EVENT LOG"=w3237:string)  [unwired: 8 in, 1 out]
                        n2194 = local write "EVENT LOG"(w3237) -> ()
                      }
                      frame #6 {
                        n2195 = Wait (ms)(milliseconds to wait=u32 50) -> ()  [unwired: 1 out]
                      }
                      frame #7 {
                        n2196 = local read "Batch Ref Num :"() -> (w3240:string)
                        n2197 = Concatenate Strings("Batch Ref No :" ("Content"), w3240) -> (w3241:string)
                        n2198 = local read "EVENT LOG"() -> (w3244:string)
                        n2199 = call "Event Log.vi"("Content"=w3241, "EVENT LOG"=w3244) -> ("EVENT LOG"=w3243:string)  [unwired: 8 in, 1 out]
                        n2200 = local write "EVENT LOG"(w3243) -> ()
                      }
                      frame #8 {
                        n2201 = Wait (ms)(milliseconds to wait=u32 50) -> ()  [unwired: 1 out]
                      }
                      frame #9 {
                        n2202 = local read "tested by"() -> (w3246:string)
                        n2203 = Concatenate Strings("Tested By :" ("Content"), w3246) -> (w3247:string)
                        n2204 = local read "EVENT LOG"() -> (w3250:string)
                        n2205 = call "Event Log.vi"("Content"=w3247, "EVENT LOG"=w3250) -> ("EVENT LOG"=w3249:string)  [unwired: 8 in, 1 out]
                        n2206 = local write "EVENT LOG"(w3249) -> ()
                      }
                      frame #10 {
                        n2207 = Wait (ms)(milliseconds to wait=u32 50) -> ()  [unwired: 1 out]
                      }
                      frame #11 {
                        n2208 = local read "TEST STANDARD"() -> (w3253:T3)
                        n2209 = case shown="\"ASTM D6079\", Default" w3253 {
                          tunnel: ["ASTM D6079" "ISO 12156" "CEC F-096-A-06" "Custom"] -> w3252
                          frame "ASTM D6079", Default {
                          }
                          frame "ISO 12156" {
                          }
                          frame "CEC F-096-A-06" {
                          }
                          frame "Custom" {
                          }
                        }
                        n2210 = Concatenate Strings("Test Standard :" ("Content"), w3252) -> (w3254:string)
                        n2211 = local read "EVENT LOG"() -> (w3257:string)
                        n2212 = call "Event Log.vi"("Content"=w3254, "EVENT LOG"=w3257) -> ("EVENT LOG"=w3256:string)  [unwired: 8 in, 1 out]
                        n2213 = local write "EVENT LOG"(w3256) -> ()
                      }
                      frame #12 {
                        n2214 = Wait (ms)(milliseconds to wait=u32 50) -> ()  [unwired: 1 out]
                      }
                      frame #13 {
                        n2215 = local read "Fuel Discription :"() -> (w3263:string)
                        n2216 = Concatenate Strings("Fuel Description :" ("Content"), w3263) -> (w3264:string)
                        n2217 = local read "EVENT LOG"() -> (w3267:string)
                        n2218 = call "Event Log.vi"("Content"=w3264, "EVENT LOG"=w3267) -> ("EVENT LOG"=w3266:string)  [unwired: 8 in, 1 out]
                        n2219 = local write "EVENT LOG"(w3266) -> ()
                      }
                      frame #14 {
                        n2220 = Wait (ms)(milliseconds to wait=u32 50) -> ()  [unwired: 1 out]
                      }
                      frame #15 {
                        n2221 = local read "Remarks :"() -> (w3269:string)
                        n2222 = Concatenate Strings("Remarks :" ("Content"), w3269) -> (w3270:string)
                        n2223 = local read "EVENT LOG"() -> (w3273:string)
                        n2224 = call "Event Log.vi"("Content"=w3270, "EVENT LOG"=w3273) -> ("EVENT LOG"=w3272:string)  [unwired: 8 in, 1 out]
                        n2225 = local write "EVENT LOG"(w3272) -> ()
                      }
                      frame #16 {
                        n2226 = Wait (ms)(milliseconds to wait=u32 50) -> ()  [unwired: 1 out]
                      }
                      frame #17 {
                        n2227 = local read "Operator ID"() -> (w3275:string)
                        n2228 = Concatenate Strings("Operator ID :" ("Content"), w3275) -> (w3277:string)
                        n2229 = local read "EVENT LOG"() -> (w3279:string)
                        n2230 = call "Event Log.vi"("Content"=w3277, "EVENT LOG"=w3279) -> ("EVENT LOG"=w3278:string)  [unwired: 8 in, 1 out]
                        n2231 = local write "EVENT LOG"(w3278) -> ()
                      }
                      frame #18 {
                        n2232 = Wait (ms)(milliseconds to wait=u32 50) -> ()  [unwired: 1 out]
                      }
                      frame #19 {
                        n2233 = disable-structure shown="Disabled" {
                          frame Disabled {
                            n2234 = local read "EVENT LOG"() -> (w3283:string)
                            n2235 = call "Event Log.vi"("Content"="Test Parameter", "EVENT LOG"=w3283) -> ("EVENT LOG"=w3282:string)  [unwired: 8 in, 1 out]
                            n2236 = local write "EVENT LOG"(w3282) -> ()
                          }
                          frame Enabled {
                          }
                        }
                      }
                      frame #20 {
                        n2237 = Wait (ms)(milliseconds to wait=u32 50) -> ()  [unwired: 1 out]
                      }
                      frame #21 {
                        n2238 = local read "Set Hz"() -> (w3287:dbl)
                        n2239 = Number To Fractional String(number=w3287, precision (6)=i16 2) -> (F-format string=w3286:string)  [unwired: 2 in]
                        n2240 = Concatenate Strings("Set Frequency [Hz] :" ("Content"), w3286) -> (w3289:string)
                        n2241 = local read "EVENT LOG"() -> (w3291:string)
                        n2242 = call "Event Log.vi"("Content"=w3289, "EVENT LOG"=w3291) -> ("EVENT LOG"=w3290:string)  [unwired: 8 in, 1 out]
                        n2243 = local write "EVENT LOG"(w3290) -> ()
                      }
                      frame #22 {
                        n2244 = Wait (ms)(milliseconds to wait=u32 50) -> ()  [unwired: 1 out]
                      }
                      frame #23 {
                        n2245 = local read "NORMAL LOAD"() -> (w3294:dbl)
                        n2246 = Number To Fractional String(number=w3294, precision (6)=i16 2) -> (F-format string=w3295:string)  [unwired: 2 in]
                        n2247 = Concatenate Strings("Applied Load [grams] :" ("Content"), w3295) -> (w3297:string)
                        n2248 = local read "EVENT LOG"() -> (w3299:string)
                        n2249 = call "Event Log.vi"("Content"=w3297, "EVENT LOG"=w3299) -> ("EVENT LOG"=w3298:string)  [unwired: 8 in, 1 out]
                        n2250 = local write "EVENT LOG"(w3298) -> ()
                      }
                      frame #24 {
                        n2251 = Wait (ms)(milliseconds to wait=u32 50) -> ()  [unwired: 1 out]
                      }
                      frame #25 {
                        n2252 = local read "Set Strk"() -> (w3302:dbl)
                        n2253 = Number To Fractional String(number=w3302, precision (6)=i16 2) -> (F-format string=w3303:string)  [unwired: 2 in]
                        n2254 = Concatenate Strings("Set Stroke [mm] :" ("Content"), w3303) -> (w3305:string)
                        n2255 = local read "EVENT LOG"() -> (w3307:string)
                        n2256 = call "Event Log.vi"("Content"=w3305, "EVENT LOG"=w3307) -> ("EVENT LOG"=w3306:string)  [unwired: 8 in, 1 out]
                        n2257 = local write "EVENT LOG"(w3306) -> ()
                      }
                      frame #26 {
                        n2258 = Wait (ms)(milliseconds to wait=u32 50) -> ()  [unwired: 1 out]
                      }
                      frame #27 {
                        n2259 = local read "Set Temp"() -> (w3310:dbl)
                        n2260 = Number To Fractional String(number=w3310, precision (6)=i16 2) -> (F-format string=w3311:string)  [unwired: 2 in]
                        n2261 = Concatenate Strings("Set Temperature [deg C] :" ("Content"), w3311) -> (w3313:string)
                        n2262 = local read "EVENT LOG"() -> (w3315:string)
                        n2263 = call "Event Log.vi"("Content"=w3313, "EVENT LOG"=w3315) -> ("EVENT LOG"=w3314:string)  [unwired: 8 in, 1 out]
                        n2264 = local write "EVENT LOG"(w3314) -> ()
                      }
                      frame #28 {
                        n2265 = Wait (ms)(milliseconds to wait=u32 50) -> ()  [unwired: 1 out]
                      }
                      frame #29 {
                        n2266 = local read "Set Rh"() -> (w3318:dbl)
                        n2267 = Number To Fractional String(number=w3318, precision (6)=i16 2) -> (F-format string=w3319:string)  [unwired: 2 in]
                        n2268 = Concatenate Strings("Set Humidity [%RH] :" ("Content"), w3319) -> (w3321:string)
                        n2269 = local read "EVENT LOG"() -> (w3323:string)
                        n2270 = call "Event Log.vi"("Content"=w3321, "EVENT LOG"=w3323) -> ("EVENT LOG"=w3322:string)  [unwired: 8 in, 1 out]
                        n2271 = local write "EVENT LOG"(w3322) -> ()
                      }
                      frame #30 {
                        n2272 = Wait (ms)(milliseconds to wait=u32 50) -> ()  [unwired: 1 out]
                      }
                      frame #31 {
                        n2273 = local read "test time"() -> (w3326:dbl)
                        n2274 = Number To Fractional String(number=w3326, precision (6)=i16 1) -> (F-format string=w3327:string)  [unwired: 2 in]
                        n2275 = Concatenate Strings("Test Duration [mins] :" ("Content"), w3327) -> (w3329:string)
                        n2276 = local read "EVENT LOG"() -> (w3331:string)
                        n2277 = call "Event Log.vi"("Content"=w3329, "EVENT LOG"=w3331) -> ("EVENT LOG"=w3330:string)  [unwired: 8 in, 1 out]
                        n2278 = local write "EVENT LOG"(w3330) -> ()
                      }
                      frame #32 {
                        w3332 = dbl[] [] ("History Data")
                        w3333 = cluster{"y":dbl, dbl, "y":dbl}[] [] ("History Data")
                        w3334 = FALSE ("Visible")
                        n2279 = property on="Stroke ( mm )" class="WFChart (strict)"("History Data"=w3333) -> ()  [unwired: 2 in, 2 out]
                        n2280 = property on="Humidity ( %RH )" class="WFChart (strict)"("History Data"=w3332) -> ()  [unwired: 2 in, 2 out]
                        n2281 = property on="Temperature ( Deg C )" class="WFChart (strict)"("History Data"=w3332) -> ()  [unwired: 2 in, 2 out]
                        n2282 = property on="Electrical Contact Resistance ( % )" class="WFChart (strict)"("History Data"=w3332) -> ()  [unwired: 2 in, 2 out]
                        n2283 = property on="Coefficient of Friction" class="WFChart (strict)"("History Data"=w3332) -> ()  [unwired: 2 in, 2 out]
                        n2284 = property on="Frictional Force ( N )" class="WFChart (strict)"("History Data"=w3332) -> ()  [unwired: 2 in, 2 out]
